vi "Stop Core.vi"(10 "final error code":i32, 11 "RDS Router Actor in":refnum<class "RDS Router Actor.lvclass">) -> (3 "RDS Router Actor out":refnum<class "RDS Router Actor.lvclass">)   [LabVIEW 2015]
doc: "(<B>Filename</B>: Actor Framework.lvlib:Actor.lvclass:Stop Core.vi)\n\nDefines what the actor does before it stops. Use the <B>final error code</B> input to determine whether the actor shut down in response to an error.\n\nBy default, this method does nothing. A descendant class may override it to define behavior, such as shutting down any processes the actor initiated in its override of the Actor Core method."
uses:
  RDS Router Actor.lvclass
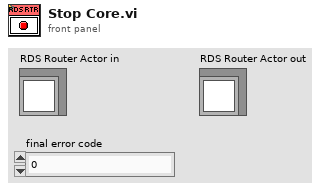
[diagram p1: front panel]
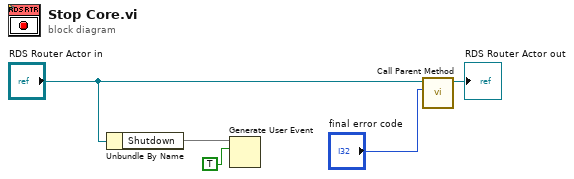
[diagram p0: block diagram]
diagram:
  n1 = Unbundle By Name("RDS Router Actor in") -> ("Shutdown"=w1)
  n2 = Generate User Event(user event=w1, event data cluster=TRUE ("event data")) -> ()  [unwired: 2 in, 2 out]
  n3 = call-parent "Call Parent Method"("final error code"="final error code", "Monitored Actor in"="RDS Router Actor in") -> ("Monitored Actor out"=→"RDS Router Actor out":refnum<class "RDS Router Actor.lvclass">)  [unwired: 9 in]
